vi "demo01_加法.vi"() -> ()   [LabVIEW 2017]
panel:
  out "c":dbl
  in  "b":dbl
  in  "a":dbl
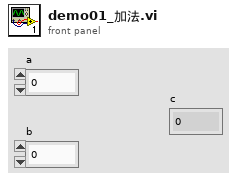
[diagram p1: front panel]
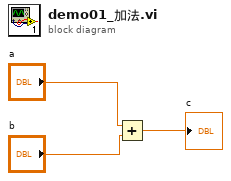
[diagram p0: block diagram]
diagram:
  n1 = Add(x="a", y="b") -> (x+y=→"c":dbl)
